vi "RIS.vi"(2 "Run uninterrupted?":bool, 3 "Device Category IN:":string(combo)="Short Strip" caption="Device Category:", 4 "Batch No.:":string, 5 "Wafer Serial No.:":string, 6 "Sensor Serial No.:":string) -> (0 "Done!":bool)   [LabVIEW 2018]
doc: "Performs Ris measurements according to ATLAS ITk Quality Control Specifications."
uses:
  <vilib>/Analysis/6fits.llb/Curve Fitting Criteria.ctl
  general_VIs/globals/QC_MeasurementSetup.vi
  general_VIs/globals/QC_RunInformation.vi
  InstrControl/InstrumentSetup.vi
  InstrControl/Switching/Switching.lvclass
  InstrControl/SupplyControl/SupplyControl.lvclass
  InstrControl/MultimeterControl/MultimeterControl.lvclass
  InstrControl/ArduinoControl/ArduinoControl.lvclass
  <vilib>/Analysis/NI_AALBase.lvlib
  InstrControl/InstrControl.lvclass
  <vilib>/Analysis/NI_AALPro.lvlib
panel:
  out "Ris":dbl[](array[numeric]) caption="Ris [MOhm]"
  out "Volts":dbl[](array[numeric]) caption="Volts [V]"
  out "Current":dbl[](array[numeric]) caption="Current [nA]"
  in  "No. of readouts":i32=5
  out "Risgraph":cluster{dbl[], dbl[]}(graph)
  out "Vigraph":cluster{i32[], dbl[]}[](graph)
  out "Imgraph":cluster{i32[], dbl[]}[](graph)
  out "Initial volts [V]":dbl format="%.1f"
  out "Final volts [V]":dbl=-700.0 format="%.1f"
  out "step [V]":dbl=10.0 format="%.1f"
  out "step interval [s]":u32=10
  out "Temp.":dbl[](array[numeric]) caption="Temp. [°C]" format="%#.2f"
  out "RH":dbl[](array[numeric]) caption="RH [%]" format="%#.2f"
  out "positive ramp?":bool
  out "Tab Control":enum32{"Ris Setup", "Ris Scan"}(tab)
  in  "Voltmeter":string(combo)="Keithley 2410"
  in  "Ris SMU":string(combo)="Keithley 2410"
  in  "Current \nLimit \n[µA]":dbl=1000.0 min=0.0001 format="%.3f"
  in  "Set\ncurrent\nlimit?":bool
  in  "Temperature":enum16{"Read Arduino", "Enter manually"}(ring)
  in  "Ris Supply":string(combo)="Keithley 2410"
  in  "User:":string(combo)="Christoph"
  in  "Configurations":bool
  in  "Manufacturer:":string(combo)="Hamamatsu"
  in  "Quit":bool
  in  "Continue":bool
  in  "abort":bool
  out "Device Category:":string
  out "Batch:":string
  out "Current Volts:":dbl format="%.2f"
  in  "quit (no save)":bool
  in  "Quit & Save":bool
  out "Bias On/Off:":bool
  out "STATUS 1":string
  out "Initiated:":string
  out "Sensor No.:":string
  out "No of steps":u32
  out "Current reading No.":u32
  out "Last reading at:":string
  out "Ris SMU Current [nA]":dbl[][][](array[numeric])
  out "Ris induced Voltage [V]":dbl[][][](array[numeric])
  # "University of\nCambridge"
  # "Strip Sensor QC: inter-strip Resistance"
  # "Ris Scan parameters:"
  # "Last 5 readings:"
  # "n-4"
  # "n-3"
  # "n-2"
  # "n-1"
  # "n"
  # "DUT & Test Description"
  # "Hardware"
  # "DUT & Test Description:"
  # "Current status:"
  # "Rdg No:"
  # "out of"
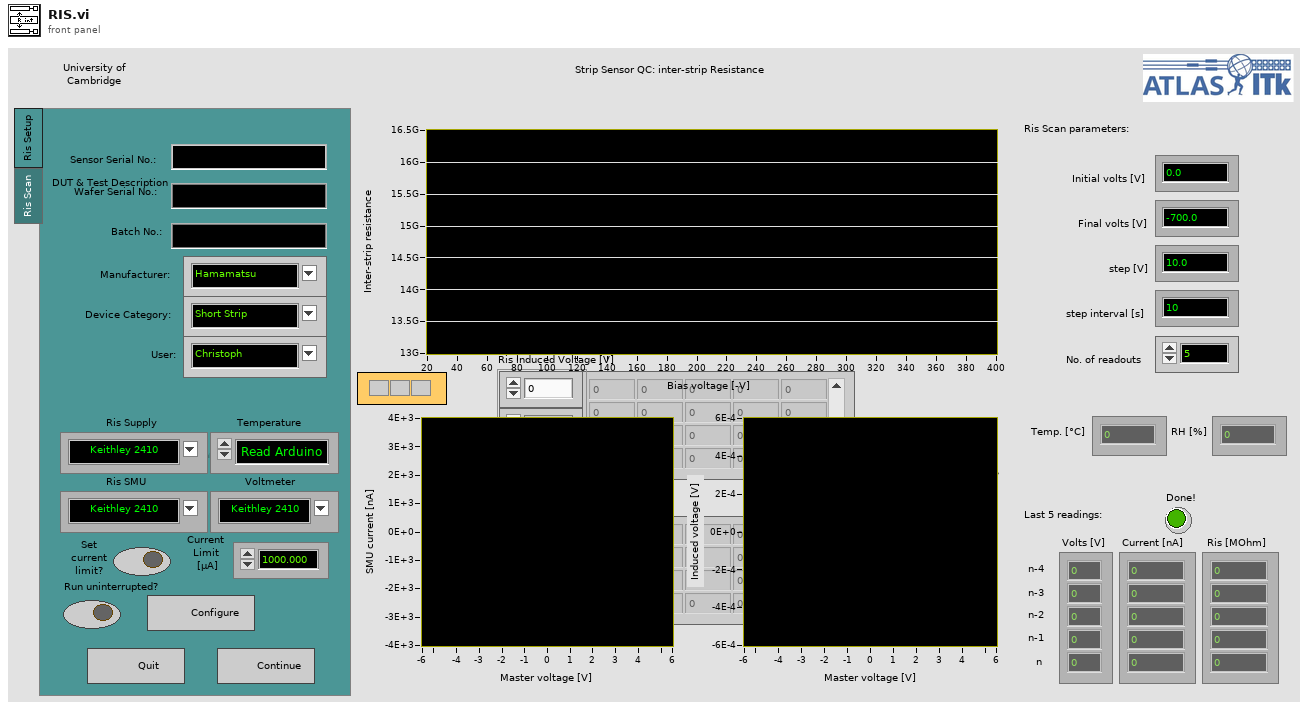
[diagram p1: front panel]
types:
  T1 = enum16{"Supply", "LCR", "Multimeter", "Switching"}
  T2 = enum16{"Reset", "Read Array", "Read Element", "Write Element", "Write Array", "Add Element", "Add Array"}
  T3 = enum16{"Reset", "Ground", "Striptest SMU", "Striptest LCR", "IV", "CV", "Interstrip Cap", "Interstrip Res"}
  T4 = enum32{"IV", "CV", "Stability", "Striptest", "Cis", "Ris", "PTP"}
  T5 = cluster{"Sensor Serial No.:":string, "Wafer Serial No.:":string, "Batch:":string, "Manufacturer:":string, "Device Category:":string, "Database Serial No.:":string, "Date Initiated:":string, "Time Initiated:":string, "Test":string, "Instruments used:":string, "Probeplan used:":string, "End of Run comment:":string, "User:":string}
  T6 = cluster{"Institute":string, "Manufacturers":string[], "Devices":string[], "Serialnumbers Lookup DB":string, "Data directory":string, "Backup & screenshot directory":string, "List of known users":string[], "Measurement switch not used":bool, "Measurement Switch":string, "DUT Switch":string}
  T7 = cluster{"Bias Supply":refnum<class "SupplyControl.lvclass">, "SMU":refnum<class "SupplyControl.lvclass">, "Multimeter":refnum<class "MultimeterControl.lvclass">, "Initial Voltage [V]":dbl, "Final Voltage [V]":dbl, "Step Size [V]":dbl, "Step Interval [s]":i32, "Number Of Steps":u32, "Ramp down steps [V]":dbl, "Ramp down Interval [s]":i32, "Set Current Limit?":bool, "Current Limit [µA]":dbl, "Temperature Readout":enum16{"Read Arduino", "Enter manually"}, "Arduino":refnum<class "ArduinoControl.lvclass">, "Supply Name":string, "SMU Name":string, "Voltmeter Name":string, "R_is Limit [MOhm]":dbl, "Switching":refnum<class "Switching.lvclass">, "Matrix used?":bool, "Matrix X Channels":cluster{"Bias Supply / SMU LO":i32, "Bias Supply / SMU HI":i32, "CV Box LO":i32, "CV Box HI":i32, "CV Box LO IN":i32, "CV Box HI IN":i32, "Volt meter LO":i32, "Volt meter HI":i32, "Mux1 C1":i32, "Mux1 C2":i32, "Mux2 C1":i32, "Mux2 C2":i32}}
  T8 = cluster{"VISA address":refnum<visa-resource-name>, "T sensor":enum16{"SHT", "DS"}, "Arduino":refnum<class "ArduinoControl.lvclass">}
  T9 = typedef "NI_AALPro.lvlib/Curve Fitting Criteria.ctl" = u16
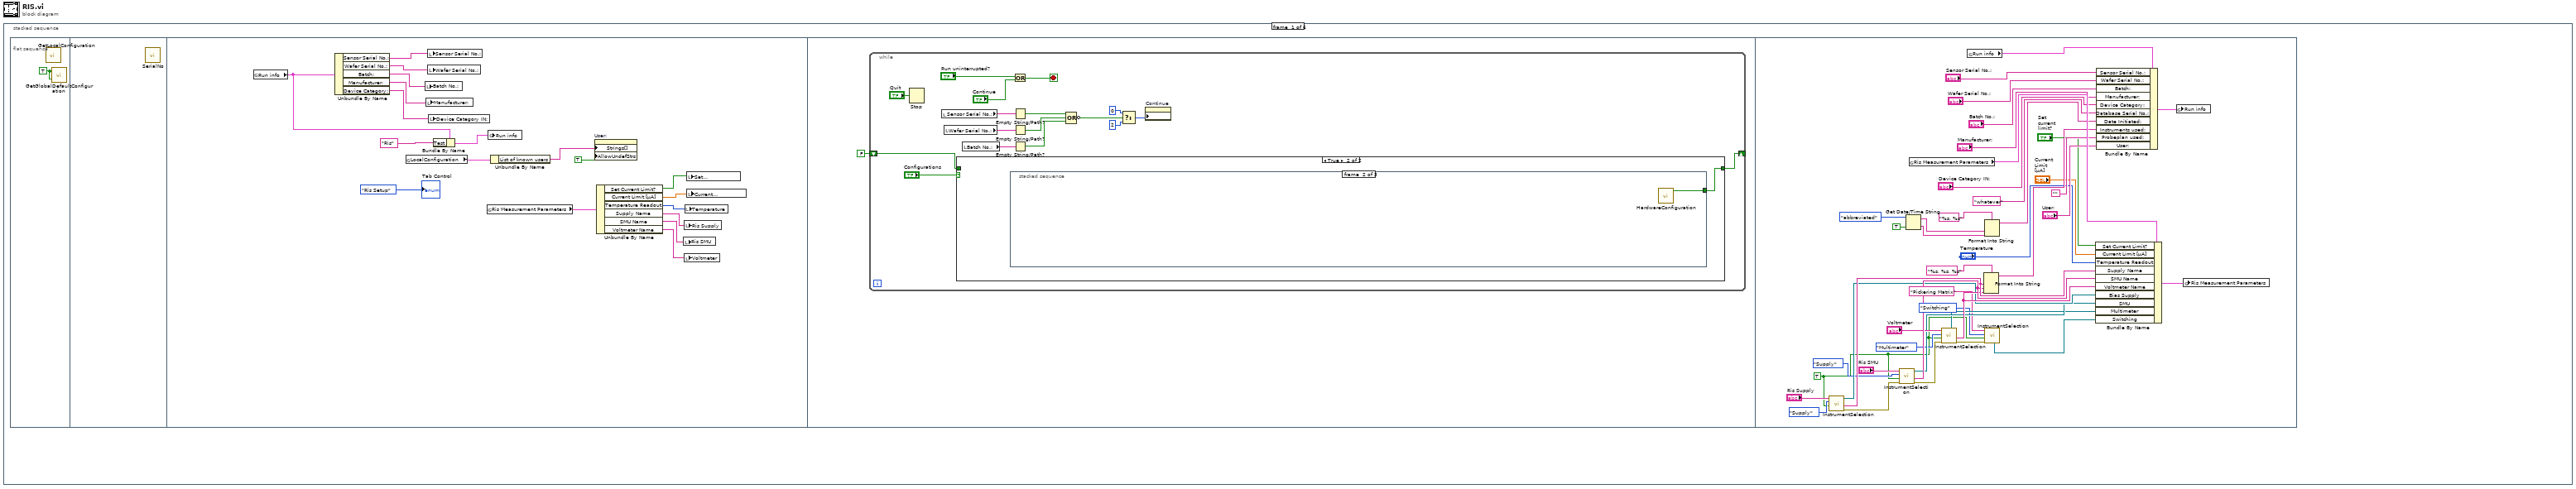
[diagram p0: block diagram]
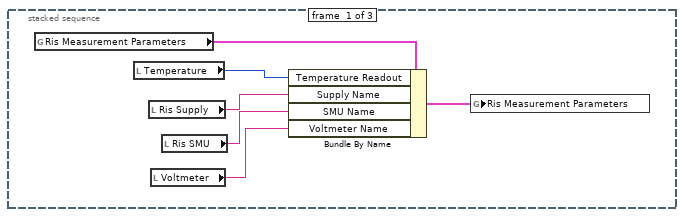
[diagram p3: hidden frame]
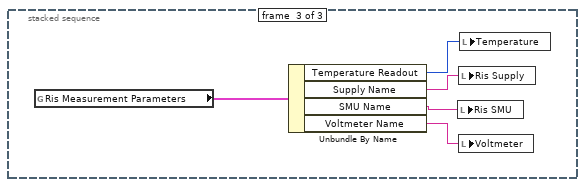
[diagram p4: hidden frame]
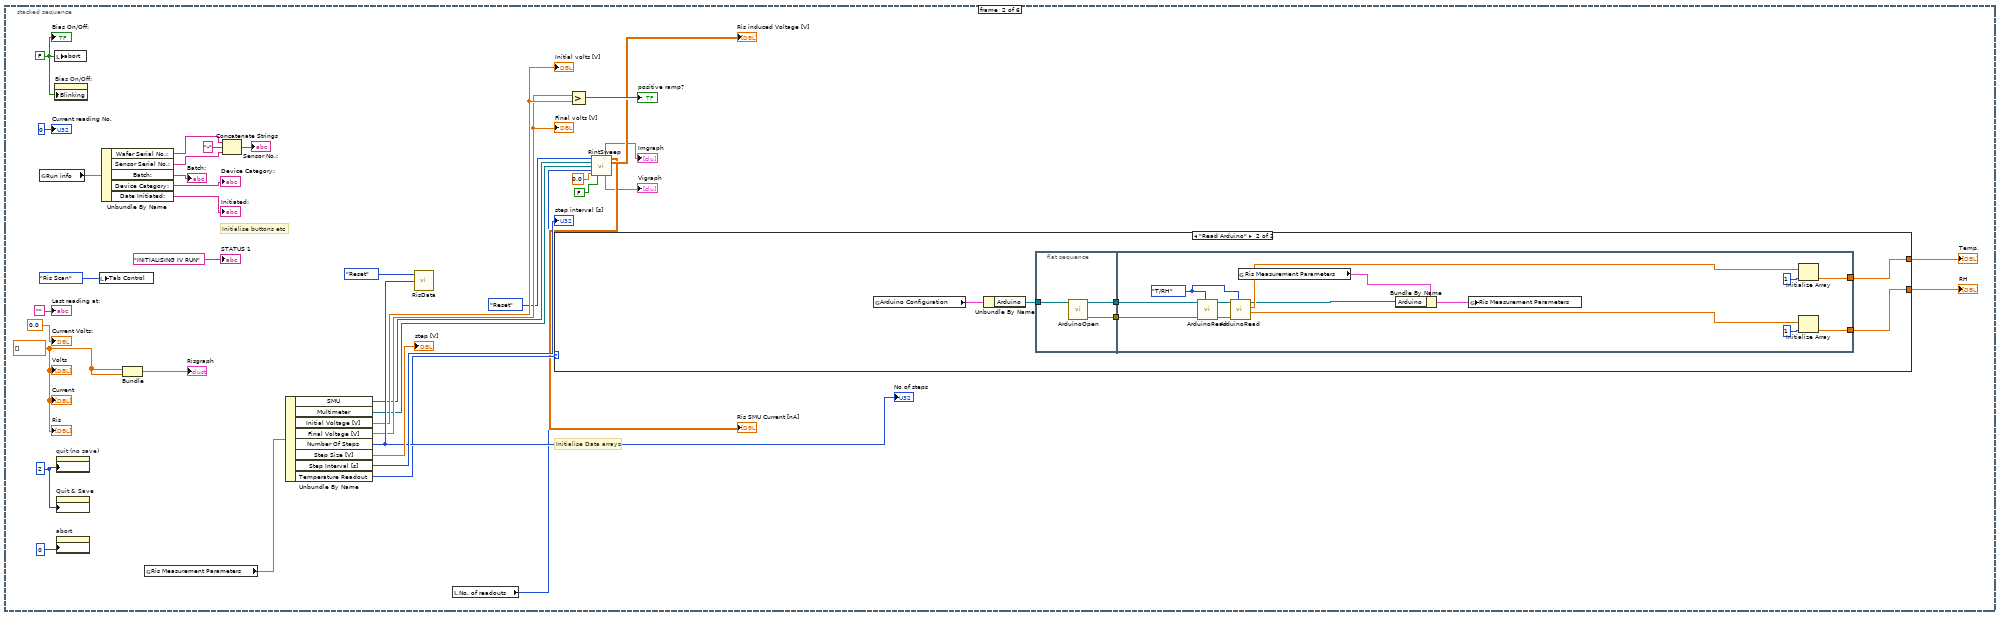
[diagram p5: hidden frame]
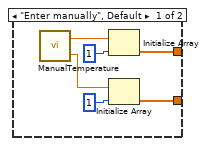
[diagram p6: hidden frame]
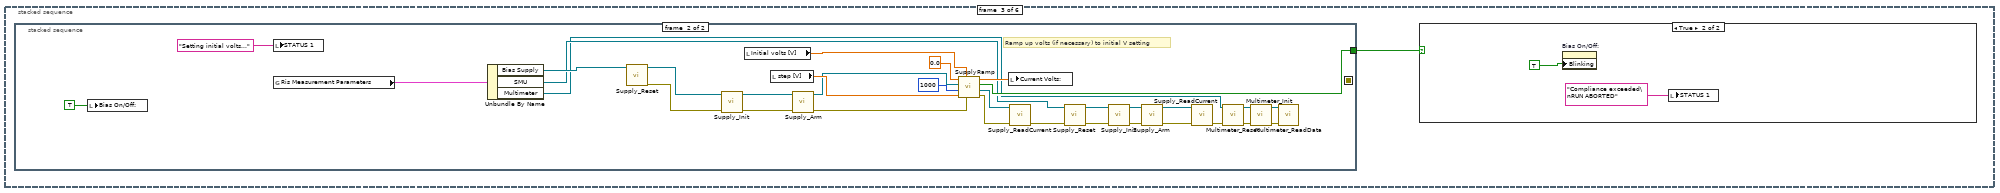
[diagram p7: hidden frame]
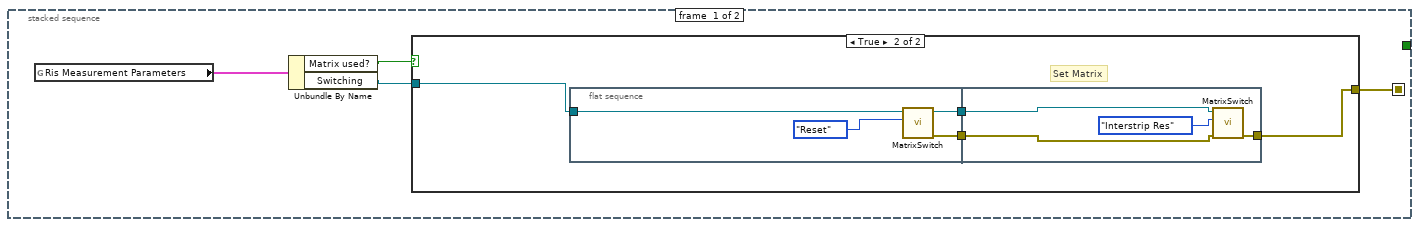
[diagram p8: hidden frame]
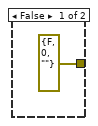
[diagram p9: hidden frame]
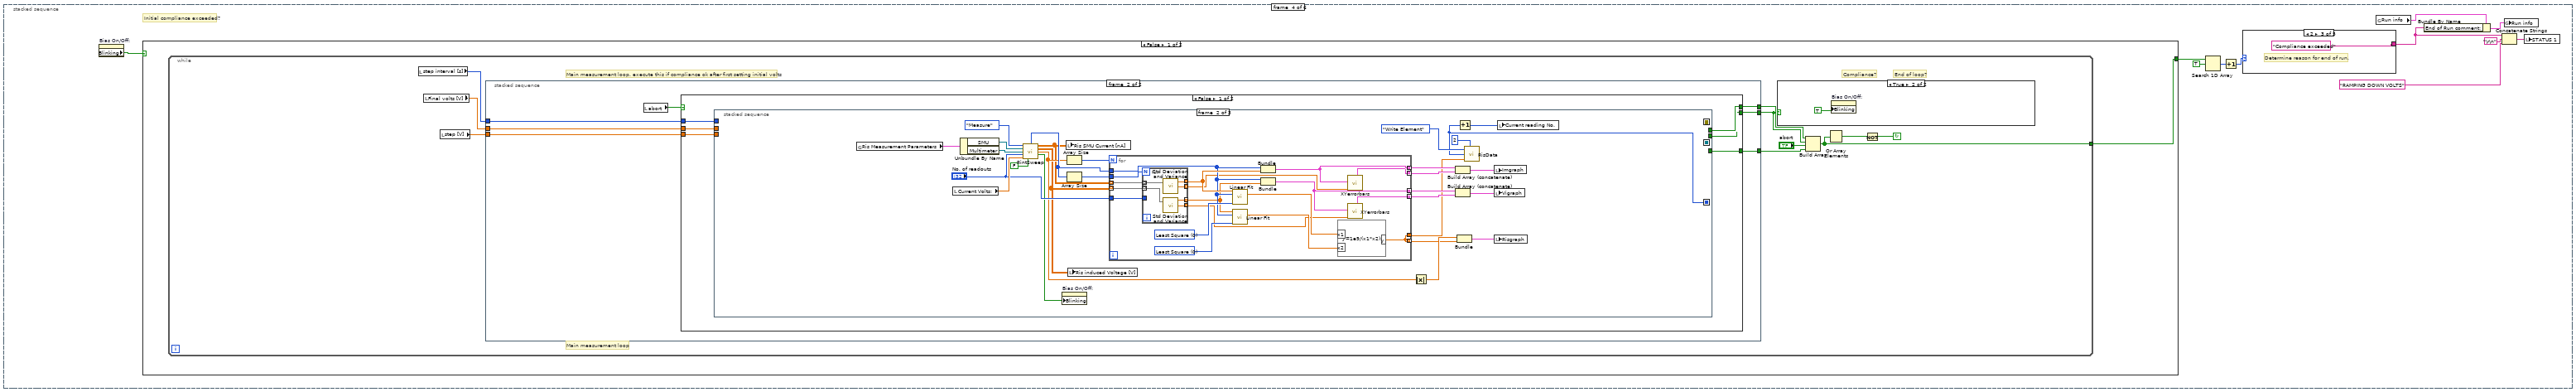
[diagram p11: hidden frame]
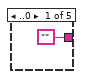
[diagram p12: hidden frame]
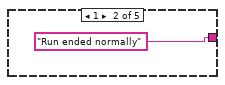
[diagram p13: hidden frame]
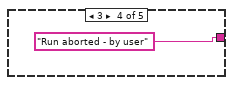
[diagram p14: hidden frame]
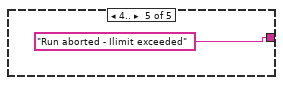
[diagram p15: hidden frame]
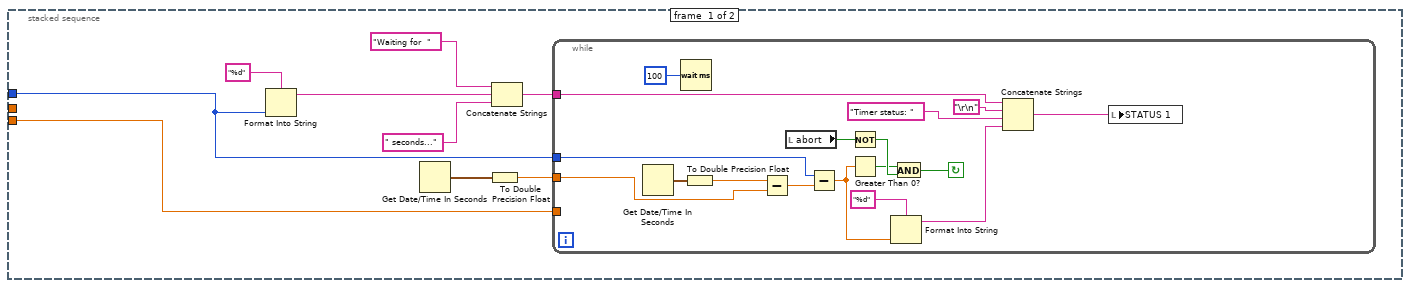
[diagram p16: hidden frame]
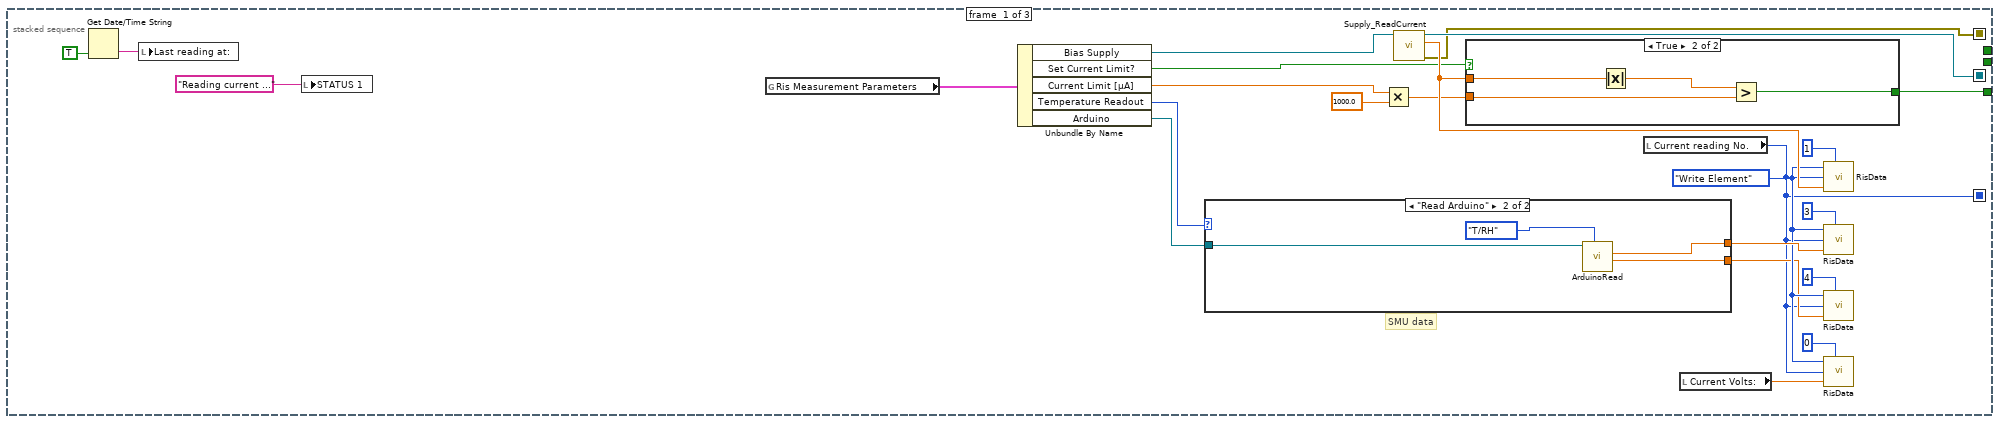
[diagram p17: hidden frame]
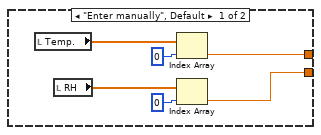
[diagram p18: hidden frame]
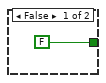
[diagram p19: hidden frame]
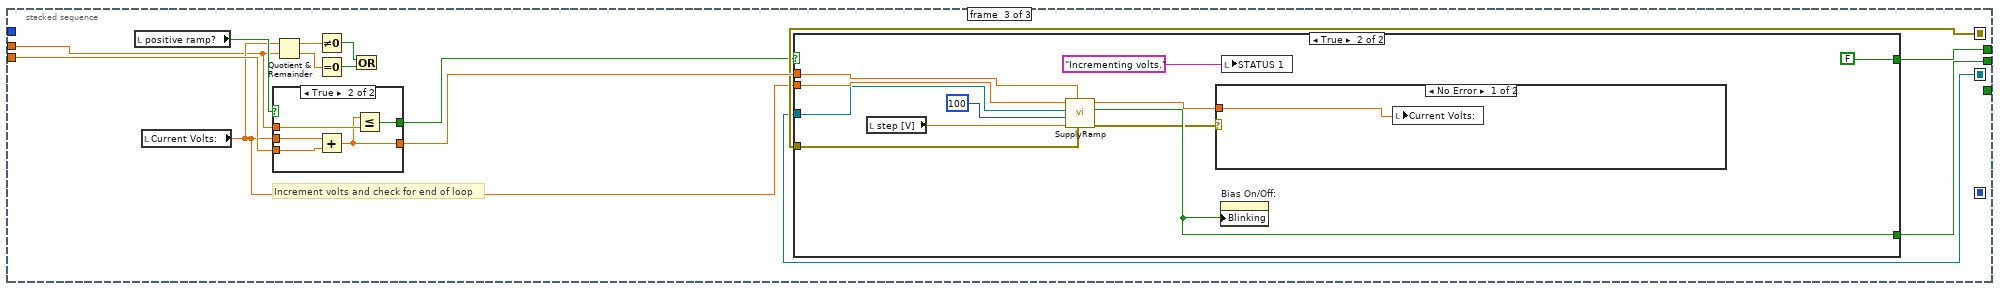
[diagram p20: hidden frame]
diagram:
  n1 = stacked-sequence {
    frame #0 {
      n2 = flat-sequence {
        frame #0 {
          w1 = TRUE
          n3 = call "GetLocalConfiguration.vi"() -> ()  [unwired: 3 in, 1 out]
          n4 = call "GetGlobalDefaultConfiguration.vi"("Run uninterrupted"=w1, "Read defaults?"=w1) -> ()  [unwired: 1 in, 1 out]
        }
        frame #1 {
          n5 = call "SerialNo.vi"() -> ()  [unwired: 5 in, 1 out]
        }
        frame #2 {
          n6 = global read "QC_RunInformation.vi" "Run info"() -> (w7:T5)
          n7 = Unbundle By Name(w7) -> ("Sensor Serial No.:"=w3:string, "Wafer Serial No.:"=w4:string, "Batch:"=w5:string, "Manufacturer:"=w2:string, "Device Category:"=w6:string)
          n8 = global read "QC_RunInformation.vi" "LocalConfiguration"() -> (w15:T6)
          n9 = local write "Batch No.:"(w5) -> ()
          n10 = local write "Manufacturer:"(w2) -> ()
          n11 = local write "Sensor Serial No.:"(w3) -> ()
          n12 = local write "Wafer Serial No.:"(w4) -> ()
          n13 = local write "Device Category IN:"(w6) -> ()
          n14 = Bundle By Name(cluster=w7, "Test"="Ris") -> (w12:T5)
          n15 = global read "QC_MeasurementSetup.vi" "Ris Measurement Parameters"() -> (w18:T7)
          n16 = global write "QC_RunInformation.vi" "Run info"(w12) -> ()
          n17 = Unbundle By Name(w15) -> ("List of known users"=w14:string[])
          n18 = property on="User:" class="CmbBox"("Strings[]"=w14, "AllowUndefStrs"=TRUE) -> ()  [unwired: 2 in, 2 out]
          n19 = Unbundle By Name(w18) -> ("Set Current Limit?"=w17:bool, "Current Limit [µA]"=w16:dbl, "Temperature Readout"=w20:enum16{"Read Arduino", "Enter manually"}, "Supply Name"=w19:string, "SMU Name"=w9:string, "Voltmeter Name"=w8:string)
          n20 = local write "Ris SMU"(w9) -> ()
          n21 = local write "Ris Supply"(w19) -> ()
          n22 = local write "Voltmeter"(w8) -> ()
          n23 = local write "Temperature"(w20) -> ()
          n24 = local write "Set\ncurrent\nlimit?"(w17) -> ()
          n25 = local write "Current \nLimit \n[µA]"(w16) -> ()
          "Tab Control" <- enum32{"Ris Setup", "Ris Scan"}."Ris Setup" ("Tab Control")
        }
        frame #3 {
          n26 = while {
            shift-right: [w26] -> _
            shift-left: FALSE -> [w25]
            stop <- w22 stop-if-true
            n27 = Stop(stop? (T)="Quit") -> ()
            n28 = local read "Sensor Serial No.:"() -> (w37:string)
            n29 = local read "Wafer Serial No.:"() -> (w36:string)
            n30 = case shown="True" "Configurations" {
              tunnel: [w39 w40] -> w26
              tunnel: w25 -> [w39 _]
              frame False {
              }
              frame True {
                n31 = stacked-sequence {
                  tunnel: [_ w47 _] -> w40
                  frame #0 {
                    n32 = global read "QC_MeasurementSetup.vi" "Ris Measurement Parameters"() -> (w46:T7)
                    n33 = local read "Temperature"() -> (w45:enum16{"Read Arduino", "Enter manually"})
                    n34 = local read "Ris Supply"() -> (w44:string)
                    n35 = local read "Voltmeter"() -> (w42:string)
                    n36 = local read "Ris SMU"() -> (w43:string)
                    n37 = Bundle By Name(cluster=w46, "Temperature Readout"=w45, "Supply Name"=w44, "SMU Name"=w43, "Voltmeter Name"=w42) -> (w41:T7)
                    n38 = global write "QC_MeasurementSetup.vi" "Ris Measurement Parameters"(w41) -> ()
                  }
                  frame #1 {
                    n39 = call "HardwareConfiguration.vi"() -> ("configured?"=w47:bool)  [unwired: 11 in]
                  }
                  frame #2 {
                    n40 = global read "QC_MeasurementSetup.vi" "Ris Measurement Parameters"() -> (w52:T7)
                    n41 = Unbundle By Name(w52) -> ("Temperature Readout"=w48:enum16{"Read Arduino", "Enter manually"}, "Supply Name"=w49:string, "SMU Name"=w50:string, "Voltmeter Name"=w51:string)
                    n42 = local write "Ris SMU"(w50) -> ()
                    n43 = local write "Ris Supply"(w49) -> ()
                    n44 = local write "Voltmeter"(w51) -> ()
                    n45 = local write "Temperature"(w48) -> ()
                  }
                }
              }
            }
            n46 = local read "Batch No.:"() -> (w28:string)
            n47 = Or(x="Run uninterrupted?", y="Continue") -> (x .or. y?=w22:bool)
            n48 = Empty String/Path?(string/path=w37) -> (empty?=w34:bool)
            n49 = Empty String/Path?(string/path=w36) -> (empty?=w35:bool)
            n50 = Empty String/Path?(string/path=w28) -> (empty?=w27:bool)
            n51 = Compound Arithmetic op=OR(w34, w35, w27) -> (invert w33:bool)
            n52 = Select(t=0, s=w33, f=2) -> (s? t:f=w30:i32)
            n53 = property on="Continue" class="Bool"("DisabledEnum"=w30) -> ()  [unwired: 2 in, 2 out]
          }
        }
        frame #4 {
          w55 = TRUE
          n54 = call "InstrumentSelection.vi"("Verify GPIB address"=w55, "Instrument type"=T1."Supply", "Instrument name IN"="Ris Supply") -> ("error out"=w62:errorcluster, "Instrument name OUT"=w70:string, "Supply"=w65:refnum<class "SupplyControl.lvclass">)  [unwired: 3 in, 3 out]
          n55 = call "InstrumentSelection.vi"("error in (no error)"=w62, "Verify GPIB address"=w55, "Instrument type"=T1."Supply", "Instrument name IN"="Ris SMU") -> ("error out"=w61:errorcluster, "Instrument name OUT"=w68:string, "Supply"=w64:refnum<class "SupplyControl.lvclass">)  [unwired: 2 in, 3 out]
          n56 = Get Date/Time String(date format (0)=enum16{"short", "long", "abbreviated"}."abbreviated", want seconds? (F)=TRUE) -> (date string=w90:string, time string=w89:string)  [unwired: 1 in]
          n57 = global read "QC_MeasurementSetup.vi" "Ris Measurement Parameters"() -> (w93:T7)
          n58 = call "InstrumentSelection.vi"("error in (no error)"=w61, "Verify GPIB address"=w55, "Instrument type"=T1."Multimeter", "Instrument name IN"="Voltmeter") -> ("error out"=w60:errorcluster, "Instrument name OUT"=w66:string, "Multimeter"=w63:refnum<class "MultimeterControl.lvclass">)  [unwired: 2 in, 3 out]
          n59 = global read "QC_RunInformation.vi" "Run info"() -> (w87:T5)
          n60 = Format Into String(format string="%s, %s, %s", w70, w68, w66) -> (resulting string=w75:string)  [unwired: 2 in, 1 out]
          n61 = Format Into String(format string="%s, %s", w90, w89) -> (resulting string=w85:string)  [unwired: 2 in, 1 out]
          n62 = call "InstrumentSelection.vi"("error in (no error)"=w60, "Verify GPIB address"=w55, "Instrument type"=T1."Switching", "Instrument name IN"="Pickering Matrix") -> ("Switching"=w54:refnum<class "Switching.lvclass">)  [unwired: 2 in, 5 out]
          n63 = Bundle By Name(cluster=w93, "Set Current Limit?"="Set\ncurrent\nlimit?", "Current Limit [µA]"="Current \nLimit \n[µA]", "Temperature Readout"="Temperature", "Supply Name"=w70, "SMU Name"=w68, "Voltmeter Name"=w66, "Bias Supply"=w65, "SMU"=w64, "Multimeter"=w63, "Switching"=w54) -> (w94:T7)
          n64 = Bundle By Name(cluster=w87, "Sensor Serial No.:"="Sensor Serial No.:", "Wafer Serial No.:"="Wafer Serial No.:", "Batch:"="Batch No.:", "Manufacturer:"="Manufacturer:", "Device Category:"="Device Category IN:", "Database Serial No.:"="whatever", "Date Initiated:"=w85, "Instruments used:"=w75, "Probeplan used:"="", "User:"="User:") -> (w86:T5)
          n65 = global write "QC_RunInformation.vi" "Run info"(w86) -> ()
          n66 = global write "QC_MeasurementSetup.vi" "Ris Measurement Parameters"(w94) -> ()
        }
      }
    }
    frame #1 {
      w100 = dbl[] []
      w122 = 2
      w121 = FALSE ("Visible")
      # "Initialise buttons etc"
      # "Initialise Data arrays"
      n67 = global read "QC_RunInformation.vi" "Run info"() -> (w132:T5)
      n68 = local write "abort"(w121) -> ()
      n69 = property on="Bias On/Off:" class="Bool (strict)"("Blinking"=w121) -> ()  [unwired: 2 in, 2 out]
      n70 = property on="quit (no save)" class="Bool"("DisabledEnum"=w122) -> ()  [unwired: 2 in, 2 out]
      n71 = property on="Quit & Save" class="Bool"("DisabledEnum"=w122) -> ()  [unwired: 2 in, 2 out]
      n72 = property on="abort" class="Bool (strict)"("DisabledEnum"=0) -> ()  [unwired: 2 in, 2 out]
      n73 = local write "Tab Control"(enum32{"Ris Setup", "Ris Scan"}."Ris Scan" ("Tab Control")) -> ()
      n74 = Unbundle By Name(w132) -> ("Wafer Serial No.:"=w113:string, "Sensor Serial No.:"=w112:string, "Batch:"=→"Batch:":string, "Device Category:"=→"Device Category:":string, "Date Initiated:"=→"Initiated:":string)
      n75 = Bundle(w100, w100) -> (→"Risgraph":cluster{dbl[], dbl[]})  [unwired: 1 in]
      n76 = global read "QC_MeasurementSetup.vi" "Ris Measurement Parameters"() -> (w115:T7)
      n77 = Concatenate Strings(w113, "-", w112) -> (→"Sensor No.:":string)
      n78 = Unbundle By Name(w115) -> ("SMU"=w96:refnum<class "SupplyControl.lvclass">, "Multimeter"=w95:refnum<class "MultimeterControl.lvclass">, "Initial Voltage [V]"=w120:dbl, "Final Voltage [V]"=w119:dbl, "Number Of Steps"=w128:u32, "Step Size [V]"=→"step [V]":dbl, "Step Interval [s]"=→"step interval [s]":i32, "Temperature Readout"=w123:enum16{"Read Arduino", "Enter manually"})
      "No of steps" <- w128
      "Initial volts [V]" <- w120
      "Final volts [V]" <- w119
      n79 = call "RisData.vi"("Action"=T2."Reset", "Array Size / Index"=w128) -> ()  [unwired: 3 in, 2 out]
      n80 = local read "No. of readouts"() -> (w98:i32)
      n81 = case shown="\"Read Arduino\"" w123 {
        tunnel: [w138 w145] -> w125
        tunnel: [w135 w144] -> w116
        frame "Enter manually", Default {
          n82 = call "ManualTemperature.vi"() -> ("Humidity [%] out"=w134:dbl, "Temperature [°C] out"=w139:dbl)
          n83 = Initialize Array(w139, 1) -> (w138:dbl[])
          n84 = Initialize Array(w134, 1) -> (w135:dbl[])
        }
        frame "Read Arduino" {
          n85 = global read "InstrumentSetup.vi" "Arduino Configuration"() -> (w141:T8)
          n86 = Unbundle By Name(w141) -> ("Arduino"=w140:refnum<class "ArduinoControl.lvclass">)
          n87 = flat-sequence {
            tunnel: [w146] -> w143
            tunnel: [w148] -> w142
            tunnel: w140 -> [w147]
            tunnel: [w162] -> w145
            tunnel: [w159] -> w144
            tunnel: w143 -> [w153]
            tunnel: w142 -> [w152]
            frame #0 {
              n88 = call "ArduinoOpen.vi"("ArduinoControl in"=w147) -> ("error out"=w148:errorcluster, "ArduinoControl out"=w146:refnum<class "ArduinoControl.lvclass">)  [unwired: 9 in]
            }
            frame #1 {
              w149 = enum16{"T/RH", "Interlock", "Edgesense"}."T/RH" ("Arduino function")
              n89 = call "ArduinoRead.vi"("Arduino function"=w149, "error in (no error)"=w152, "ArduinoControl in"=w153) -> ("error out"=w151:errorcluster, "ArduinoControl out"=w150:refnum<class "ArduinoControl.lvclass">)  [unwired: 3 in, 4 out]
              n90 = call "ArduinoRead.vi"("Arduino function"=w149, "error in (no error)"=w151, "ArduinoControl in"=w150) -> ("rel. Humidity [%]"=w157:dbl, "Temperature [°C]"=w158:dbl, "ArduinoControl out"=w156:refnum<class "ArduinoControl.lvclass">)  [unwired: 3 in, 3 out]
              n91 = global read "QC_MeasurementSetup.vi" "Ris Measurement Parameters"() -> (w155:T7)
              n92 = Bundle By Name(cluster=w155, "Arduino"=w156) -> (w154:T7)
              n93 = global write "QC_MeasurementSetup.vi" "Ris Measurement Parameters"(w154) -> ()
              n94 = Initialize Array(w158, 1) -> (w162:dbl[])
              n95 = Initialize Array(w157, 1) -> (w159:dbl[])
            }
          }
        }
      }
      "Temp." <- w125
      "RH" <- w116
      n96 = Greater?(x=w119, y=w120) -> (0:→"positive ramp?":bool)
      n97 = call "RintSweep.vi"("Action"=enum16{"Reset", "Measure"}."Reset", "MasterVoltage Supply in"=w96, "VoltmeterControl in"=w95, "No. of readouts"=w98, "Bias [V]"=0.0, "Simulated data?"=FALSE) -> ("Igraph"=→"Imgraph":cluster{i32[], dbl[]}[], "Applied Current [nA]"=→"Ris SMU Current [nA]":dbl[][][], "Induced Voltage [V]"=→"Ris induced Voltage [V]":dbl[][][], "ViGraph"=→"Vigraph":cluster{i32[], dbl[]}[])  [unwired: 2 in, 4 out]
      "STATUS 1" <- "INITIALISING IV RUN"
      "Bias On/Off:" <- w121
      "Last reading at:" <- ""
      "Current reading No." <- u32 0 ("Current reading No.")
      "Current Volts:" <- 0.0 ("Current Volts:")
      "Current" <- w100
      "Volts" <- w100
      "Ris" <- w100
    }
    frame #2 {
      n98 = stacked-sequence {
        seq-local: [w165 _] -> [_ _]
        tunnel: [_ w195] -> w163
        frame #0 {
          n99 = global read "QC_MeasurementSetup.vi" "Ris Measurement Parameters"() -> (w164:T7)
          n100 = Unbundle By Name(w164) -> ("Matrix used?"=w167:bool, "Switching"=w166:refnum<class "Switching.lvclass">)
          n101 = case shown="True" w167 {
            tunnel: w166 -> [_ w169]
            tunnel: [errorcluster {"status"=FALSE, "code"=0, "source"=""} ("error constant") w170] -> w165
            frame False {
            }
            frame True {
              # "Set Matrix"
              n102 = flat-sequence {
                tunnel: [w176] -> w172
                tunnel: [w175] -> w171
                tunnel: w169 -> [w173]
                tunnel: w172 -> [w180]
                tunnel: w171 -> [w179]
                tunnel: [w178] -> w170
                frame #0 {
                  n103 = call-dynamic "MatrixSwitch.vi"("Action"=T3."Reset", "Switching in"=w173) -> ("error out"=w176:errorcluster, "Switching out"=w175:refnum<class "Switching.lvclass">)  [unwired: 7 in, 1 out]
                }
                frame #1 {
                  n104 = call-dynamic "MatrixSwitch.vi"("error in (no error)"=w180, "Action"=T3."Interstrip Res", "Switching in"=w179) -> ("error out"=w178:errorcluster)  [unwired: 6 in, 2 out]
                }
              }
            }
          }
        }
        frame #1 {
          # "Ramp up volts (if necessary) to initial V setting"
          n105 = local write "Bias On/Off:"(TRUE ("Compliance?")) -> ()
          n106 = local write "STATUS 1"("Setting initial volts..." ("STATUS 1")) -> ()
          n107 = global read "QC_MeasurementSetup.vi" "Ris Measurement Parameters"() -> (w208:T7)
          n108 = Unbundle By Name(w208) -> ("Bias Supply"=w205:refnum<class "SupplyControl.lvclass">, "SMU"=w187:refnum<class "SupplyControl.lvclass">, "Multimeter"=w182:refnum<class "MultimeterControl.lvclass">)
          n109 = call-dynamic "Supply_Reset.vi"("SupplyControl in"=w205) -> ("error out"=w210:errorcluster, "SupplyControl out"=w212:refnum<class "SupplyControl.lvclass">)  [unwired: 9 in]
          n110 = call-dynamic "Supply_Init.vi"("error in (no error)"=w210, "SupplyControl in"=w212) -> ("error out"=w209:errorcluster, "SupplyControl out"=w211:refnum<class "SupplyControl.lvclass">)  [unwired: 8 in]
          n111 = local read "Initial volts [V]"() -> (w198:dbl)
          n112 = local read "step [V]"() -> (w199:dbl)
          n113 = call-dynamic "Supply_Arm.vi"("error in (no error)"=w209, "SupplyControl in"=w211) -> ("error out"=w197:errorcluster, "SupplyControl out"=w196:refnum<class "SupplyControl.lvclass">)  [unwired: 8 in]
          n114 = call "SupplyRamp.vi"("error in"=w197, "Requested Voltage"=w198, "Step Size"=w199, "Step Delay"=1000, "Supply IN"=w196, "Starting Voltage"=0.0) -> ("error out"=w203:errorcluster, "Supply OUT"=w204:refnum<class "SupplyControl.lvclass">, "Compliance exceeded"=w195:bool, "Current Voltage"=w202:dbl)  [unwired: 2 in]
          n115 = local write "Current Volts:"(w202) -> ()
          n116 = call-dynamic "Supply_ReadCurrent.vi"("error in (no error)"=w203, "SupplyControl in"=w204) -> ("error out"=w188:errorcluster)  [unwired: 7 in, 2 out]
          n117 = call-dynamic "Supply_Reset.vi"("error in (no error)"=w188, "SupplyControl in"=w187) -> ("error out"=w192:errorcluster, "SupplyControl out"=w194:refnum<class "SupplyControl.lvclass">)  [unwired: 8 in]
          n118 = call-dynamic "Supply_Init.vi"("error in (no error)"=w192, "SupplyControl in"=w194) -> ("error out"=w191:errorcluster, "SupplyControl out"=w193:refnum<class "SupplyControl.lvclass">)  [unwired: 8 in]
          n119 = call-dynamic "Supply_Arm.vi"("error in (no error)"=w191, "SupplyControl in"=w193) -> ("error out"=w190:errorcluster, "SupplyControl out"=w189:refnum<class "SupplyControl.lvclass">)  [unwired: 8 in]
          n120 = call-dynamic "Supply_ReadCurrent.vi"("error in (no error)"=w190, "SupplyControl in"=w189) -> ("error out"=w181:errorcluster)  [unwired: 7 in, 2 out]
          n121 = call-dynamic "Multimeter_Reset.vi"("error in (no error)"=w181, "MultimeterControl in"=w182) -> ("error out"=w183:errorcluster, "MultimeterControl out"=w184:refnum<class "MultimeterControl.lvclass">)  [unwired: 8 in]
          n122 = call-dynamic "Multimeter_Init.vi"("error in (no error)"=w183, "MultimeterControl in"=w184) -> ("error out"=w186:errorcluster, "MultimeterControl out"=w185:refnum<class "MultimeterControl.lvclass">)  [unwired: 8 in]
          n123 = call-dynamic "Multimeter_ReadData.vi"("error in (no error)"=w186, "MultimeterControl in"=w185) -> ()  [unwired: 7 in, 3 out]
        }
      }
      n124 = case shown="True" w163 {
        frame False {
        }
        frame True {
          n125 = property on="Bias On/Off:" class="Bool (strict)"("Blinking"=TRUE) -> ()  [unwired: 2 in, 2 out]
          n126 = local write "STATUS 1"("Compliance exceeded\nRUN ABORTED") -> ()
        }
      }
    }
    frame #3 {
      # "Initial compliance exceeded?"
      n127 = property on="Bias On/Off:" class="Bool (strict)"() -> ("Blinking"=w225:bool)  [unwired: 2 in, 2 out]
      n128 = case shown="False" w225 {
        tunnel: [w231 w413] -> w224
        frame False {
          n129 = while {
            tunnel: [w239] -> w231
            stop <- w240 continue-if-true
            # "Main measurement loop"
            # "End of loop?"
            # "Compliance?"
            # "Main measurement loop. execute this if compliance ok after first setting initial volts"
            n130 = local read "step interval [s]"() -> (w236:u32)
            n131 = local read "Final volts [V]"() -> (w237:dbl)
            n132 = local read "step [V]"() -> (w238:dbl)
            n133 = stacked-sequence {
              tunnel: w238 -> [w250 w274]
              tunnel: [_ w273] -> w233
              tunnel: w237 -> [_ w272]
              tunnel: w236 -> [w242 w271]
              tunnel: [_ w270] -> w235
              tunnel: [_ w268] -> w234
              frame #0 {
                n134 = Format Into String(format string="%d", w242) -> (resulting string=w247:string)  [unwired: 2 in, 1 out]
                n135 = Get Date/Time In Seconds() -> (seconds since 1Jan1904=w244:timestamp)
                n136 = To Double Precision Float(number=w244) -> (double precision float=w245:dbl)
                n137 = Concatenate Strings("Waiting for  ", w247, " seconds...") -> (w243:string)
                n138 = while {
                  tunnel: w250 -> [_]
                  tunnel: w243 -> [w255]
                  tunnel: w242 -> [w261]
                  tunnel: w245 -> [w262]
                  stop <- w263 continue-if-true
                  n139 = Get Date/Time In Seconds() -> (seconds since 1Jan1904=w254:timestamp)
                  n140 = Wait (ms)(milliseconds to wait=u32 100) -> ()  [unwired: 1 out]
                  n141 = To Double Precision Float(number=w254) -> (double precision float=w267:dbl)
                  n142 = Subtract(x=w267, y=w262) -> (x-y=w252:dbl)
                  n143 = local read "abort"() -> (w260:bool)
                  n144 = Subtract(x=w261, y=w252) -> (x-y=w251:dbl)
                  n145 = Not(x=w260) -> (.not. x?=w266:bool)
                  n146 = Greater Than 0?(x=w251) -> (x > 0?=w253:bool)
                  n147 = Format Into String(format string="%d", w251) -> (resulting string=w265:string)  [unwired: 2 in, 1 out]
                  n148 = And(x=w253, y=w266) -> (x .and. y?=w263:bool)
                  n149 = Concatenate Strings(w255, "\r\n", "Timer status: ", w265) -> (w259:string)
                  n150 = local write "STATUS 1"(w259) -> ()
                }
              }
              frame #1 {
                n151 = local read "abort"() -> (w269:bool)
                n152 = case shown="False" w269 {
                  tunnel: [w280 w410] -> w270
                  tunnel: w271 -> [w279 _]
                  tunnel: w272 -> [w278 _]
                  tunnel: [w276 w410] -> w273
                  tunnel: w274 -> [w277 _]
                  tunnel: [w275 w410] -> w268
                  frame False {
                    n153 = stacked-sequence {
                      seq-local: [w281 _ _] -> [_ w321 _]
                      seq-local: [w291 _ _] -> [_ _ w379]
                      seq-local: [w290 _ _] -> [_ _ w380]
                      tunnel: w277 -> [_ _ w385]
                      tunnel: w278 -> [_ _ w376]
                      tunnel: [_ _ w383] -> w280
                      tunnel: [_ _ w382] -> w276
                      tunnel: w279 -> [_ _ _]
                      tunnel: [w298 _ _] -> w275
                      frame #0 {
                        w293 = T2."Write Element" ("Action")
                        # "SMU data"
                        n154 = Get Date/Time String(want seconds? (F)=TRUE) -> (time string=w295:string)  [unwired: 2 in, 1 out]
                        n155 = local write "Last reading at:"(w295) -> ()
                        n156 = local write "STATUS 1"("Reading current ..." ("status")) -> ()
                        n157 = global read "QC_MeasurementSetup.vi" "Ris Measurement Parameters"() -> (w289:T7)
                        n158 = Unbundle By Name(w289) -> ("Bias Supply"=w283:refnum<class "SupplyControl.lvclass">, "Set Current Limit?"=w288:bool, "Current Limit [µA]"=w285:dbl, "Temperature Readout"=w287:enum16{"Read Arduino", "Enter manually"}, "Arduino"=w282:refnum<class "ArduinoControl.lvclass">)
                        n159 = case shown="\"Read Arduino\"" w287 {
                          tunnel: [w308 w314] -> w296
                          tunnel: [w305 w313] -> w292
                          tunnel: w282 -> [_ w312]
                          frame "Enter manually", Default {
                            n160 = local read "Temp."() -> (w310:dbl[])
                            n161 = local read "RH"() -> (w306:dbl[])
                            n162 = Index Array(array=w310, index=0) -> (element=w308:dbl)
                            n163 = Index Array(array=w306, index=0) -> (element=w305:dbl)
                          }
                          frame "Read Arduino" {
                            n164 = call "ArduinoRead.vi"("Arduino function"=enum16{"T/RH", "Interlock", "Edgesense"}."T/RH", "ArduinoControl in"=w312) -> ("rel. Humidity [%]"=w313:dbl, "Temperature [°C]"=w314:dbl)  [unwired: 4 in, 4 out]
                          }
                        }
                        n165 = Multiply(x=w285, y=1000.0) -> (x*y=w284:dbl)
                        n166 = call-dynamic "Supply_ReadCurrent.vi"("SupplyControl in"=w283) -> ("error out"=w290:errorcluster, "Current in nA"=w299:dbl, "SupplyControl out"=w291:refnum<class "SupplyControl.lvclass">)  [unwired: 8 in]
                        n167 = case shown="True" w288 {
                          tunnel: w299 -> [_ w319]
                          tunnel: w284 -> [_ w317]
                          tunnel: [FALSE w316] -> w298
                          frame False {
                          }
                          frame True {
                            n168 = Absolute Value(x=w319) -> (abs(x)=w318:dbl)
                            n169 = Greater?(x=w318, y=w317) -> (0:w316:bool)
                          }
                        }
                        n170 = local read "Current reading No."() -> (w281:u32)
                        n171 = local read "Current Volts:"() -> (w300:dbl)
                        n172 = call "RisData.vi"("Action"=w293, "Array No."=u32 1, "Array Size / Index"=w281, "Data IN"=w299) -> ()  [unwired: 1 in, 2 out]
                        n173 = call "RisData.vi"("Action"=w293, "Array No."=u32 3, "Array Size / Index"=w281, "Data IN"=w296) -> ()  [unwired: 1 in, 2 out]
                        n174 = call "RisData.vi"("Action"=w293, "Array No."=u32 4, "Array Size / Index"=w281, "Data IN"=w292) -> ()  [unwired: 1 in, 2 out]
                        n175 = call "RisData.vi"("Action"=w293, "Array No."=0, "Array Size / Index"=w281, "Data IN"=w300) -> ()  [unwired: 1 in, 2 out]
                      }
                      frame #1 {
                        n176 = global read "QC_MeasurementSetup.vi" "Ris Measurement Parameters"() -> (w340:T7)
                        n177 = local read "Current Volts:"() -> (w343:dbl)
                        n178 = Unbundle By Name(w340) -> ("SMU"=w339:refnum<class "SupplyControl.lvclass">, "Multimeter"=w338:refnum<class "MultimeterControl.lvclass">)
                        n179 = call "RintSweep.vi"("Action"=enum16{"Reset", "Measure"}."Measure", "MasterVoltage Supply in"=w339, "VoltmeterControl in"=w338, "No. of readouts"="No. of readouts", "Bias [V]"=w343, "Simulated data?"=FALSE) -> ("Sweep"=w347:i32[], "Applied Current [nA]"=w327:dbl[][][], "Induced Voltage [V]"=w328:dbl[][][], "Voltages OUT"=w330:dbl[], "Compliance exceeded?"=w337:bool)  [unwired: 2 in, 3 out]
                        n180 = property on="Bias On/Off:" class="Bool (strict)"("Blinking"=w337) -> ()  [unwired: 2 in, 2 out]
                        n181 = local write "Ris SMU Current [nA]"(w327) -> ()
                        n182 = Array Size(array=w330) -> (size(s)=w345:i32)
                        n183 = Array Size(array=w347) -> (size(s)=w346:i32)
                        n184 = local write "Ris induced Voltage [V]"(w328) -> ()
                        n185 = for {
                          N: w345 -> [_]
                          tunnel: "No. of readouts" -> [w365]
                          tunnel: w346 -> [w364]
                          tunnel: w327 -> [w363] mode=indexing
                          tunnel: w328 -> [w362] mode=indexing
                          tunnel: w347 -> [w358]
                          tunnel: [w353] -> w336 mode=indexing
                          tunnel: [w352] -> w333 mode=indexing
                          tunnel: [w354] -> w326 mode=indexing
                          tunnel: [w354] -> w322
                          tunnel: [w349] -> w335 mode=indexing
                          tunnel: [w348] -> w332 mode=indexing
                          w361 = T9 0 items=["Least Square", "Least Absolute Residual", "Bisquare"] ("method")
                          w360 = T9 0 items=["Least Square", "Least Absolute Residual", "Bisquare"] ("method")
                          n186 = for {
                            N: w364 -> [_]
                            tunnel: w365 -> [_]
                            tunnel: w363 -> [w371] mode=indexing
                            tunnel: w362 -> [w370] mode=indexing
                            tunnel: [w369] -> w359 mode=indexing
                            tunnel: [w368] -> w357 mode=indexing
                            tunnel: [w367] -> w350 mode=indexing
                            tunnel: [w366] -> w351 mode=indexing
                            n187 = call <vilib>:"Std Deviation and Variance.vi"("X"=w371) -> ("mean"=w369:dbl, "standard deviation"=w367:dbl)  [unwired: 1 in, 1 out]
                            n188 = call <vilib>:"Std Deviation and Variance.vi"("X"=w370) -> ("mean"=w368:dbl, "standard deviation"=w366:dbl)  [unwired: 1 in, 1 out]
                          }
                          n189 = call <vilib>:"Linear Fit.vi"("Y"=w359, "X"=w358, "method"=w361) -> ("slope"=w355:dbl)  [unwired: 8 in, 4 out]
                          n190 = call <vilib>:"Linear Fit.vi"("Y"=w357, "X"=w358, "method"=w360) -> ("slope"=w356:dbl)  [unwired: 8 in, 4 out]
                          n191 = Bundle("Sweep"=w358, w359) -> (w353:cluster{"Sweep":i32[], dbl[]})  [unwired: 1 in]
                          n192 = Bundle("Sweep"=w358, w357) -> (w352:cluster{"Sweep":i32[], dbl[]})  [unwired: 1 in]
                          n193 = formula code="y=1e9/(x1*x2);"("x1"=w355, "x2"=w356) -> ("y"=w354:dbl)
                          n194 = call "XYerrorbars.vi"("XY plot"=w353, "Yerror"=w350) -> ("Y error bars"=w349:cluster{dbl[], dbl[]})  [unwired: 6 in, 2 out]
                          n195 = call "XYerrorbars.vi"("XY plot"=w352, "Yerror"=w351) -> ("Y error bars"=w348:cluster{dbl[], dbl[]})  [unwired: 6 in, 2 out]
                        }
                        n196 = Absolute Value(x=w330) -> (abs(x)=w329:dbl[])
                        n197 = Build Array (concatenate)(w336, w335) -> (w334:cluster{"Sweep":dbl[], dbl[]}[])
                        n198 = Build Array (concatenate)(w333, w332) -> (w331:cluster{"Sweep":dbl[], dbl[]}[])
                        n199 = Bundle(w329, w326) -> (w325:cluster{dbl[], dbl[]})  [unwired: 1 in]
                        n200 = Increment(x=w321) -> (x+1=w320:u32)
                        n201 = call "RisData.vi"("Action"=T2."Write Element", "Array No."=2, "Array Size / Index"=w321, "Data IN"=w322) -> ()  [unwired: 1 in, 2 out]
                        n202 = local write "Imgraph"(w334) -> ()
                        n203 = local write "Vigraph"(w331) -> ()
                        n204 = local write "Risgraph"(w325) -> ()
                        n205 = local write "Current reading No."(w320) -> ()
                      }
                      frame #2 {
                        # "Increment volts and check for end of loop"
                        n206 = local read "positive ramp?"() -> (w381:bool)
                        n207 = local read "Current Volts:"() -> (w377:dbl)
                        n208 = case shown="True" w381 {
                          tunnel: w376 -> [w388 w392]
                          tunnel: w385 -> [w389 w395]
                          tunnel: [w387 w394] -> w372
                          tunnel: [w386 w391] -> w384
                          tunnel: w377 -> [w390 w393]
                          frame False {
                            n209 = Subtract(x=w390, y=w389) -> (x-y=w386:dbl)
                            n210 = Greater Or Equal?(x=w386, y=w388) -> (x >= y?=w387:bool)
                          }
                          frame True {
                            n211 = Add(x=w393, y=w395) -> (x+y=w391:dbl)
                            n212 = Less Or Equal?(x=w391, y=w392) -> (x <= y?=w394:bool)
                          }
                        }
                        n213 = Quotient & Remainder(x=w377, y=w376) -> (x-y*floor(x/y)=w378:dbl, floor(x/y)=w375:dbl)
                        n214 = Not Equal To 0?(x=w378) -> (x != 0?=w373:bool)
                        n215 = Equal To 0?(x=w375) -> (x = 0?=w374:bool)
                        n216 = Or(x=w373, y=w374) -> ()  [unwired: 1 out]
                        n217 = case shown="True" w372 {
                          tunnel: w384 -> [_ w406]
                          tunnel: [TRUE FALSE] -> w383
                          tunnel: [FALSE w407] -> w382
                          tunnel: w377 -> [_ w404]
                          tunnel: w380 -> [_ w403]
                          tunnel: w379 -> [_ w402]
                          frame False {
                          }
                          frame True {
                            n218 = local read "step [V]"() -> (w400:dbl)
                            n219 = call "SupplyRamp.vi"("error in"=w403, "Requested Voltage"=w406, "Step Size"=w400, "Step Delay"=100, "Supply IN"=w402, "Starting Voltage"=w404) -> ("error out"=w398:errorcluster, "Compliance exceeded"=w407:bool, "Current Voltage"=w401:dbl)  [unwired: 2 in, 1 out]
                            n220 = case shown="No Error" w398 {
                              tunnel: w401 -> [w409 _]
                              frame No Error {
                                n221 = local write "Current Volts:"(w409) -> ()
                              }
                              frame Error {
                              }
                            }
                            n222 = property on="Bias On/Off:" class="Bool (strict)"("Blinking"=w407) -> ()  [unwired: 2 in, 2 out]
                            n223 = local write "STATUS 1"("Incrementing volts.") -> ()
                          }
                        }
                      }
                    }
                  }
                  frame True {
                    w410 = FALSE
                  }
                }
              }
            }
            n224 = case shown="True" w233 {
              frame False {
              }
              frame True {
                n225 = property on="Bias On/Off:" class="Bool (strict)"("Blinking"=TRUE) -> ()  [unwired: 2 in, 2 out]
              }
            }
            n226 = Build Array(w235, w233, "abort", w234) -> (w239:bool[])
            n227 = Or Array Elements(Boolean array=w239) -> (logical OR=w241:bool)
            n228 = Not(x=w241) -> (.not. x?=w240:bool)
          }
        }
        frame True {
          w412 = FALSE
          # "compliance was exceeded when first voltage applied."
          # "Flag compliance as reason for end of run"
          n229 = local write "STATUS 1"("Run aborted - compliance exceeded.") -> ()
          n230 = Build Array(w412, TRUE, w412, w412) -> (w413:bool[])
        }
      }
      n231 = Search 1D Array(1D array=w224, element=TRUE) -> (index of element=w222:i32)  [unwired: 1 in]
      n232 = Increment(x=w222) -> (x+1=w221:i32)
      n233 = case shown="2" w221 {
        tunnel: ["" "Run ended normally" "Compliance exceeded" "Run aborted - by user" "Run aborted - Ilimit exceeded"] -> w216
        frame ..0 {
        }
        frame 1 {
        }
        frame 2 {
          # "Determine reason for end of run."
        }
        frame 3 {
        }
        frame 4.. {
        }
      }
      n234 = global read "QC_RunInformation.vi" "Run info"() -> (w220:T5)
      n235 = Bundle By Name(cluster=w220, "End of Run comment:"=w216) -> (w215:T5)
      n236 = Concatenate Strings(w216, "\r\n", "RAMPING DOWN VOLTS") -> (w219:string)
      n237 = global write "QC_RunInformation.vi" "Run info"(w215) -> ()
      n238 = local write "STATUS 1"(w219) -> ()
    }
    frame #4 {
      n239 = stacked-sequence {
        frame #0 {
          # "Tie up loose ends. Set volts to zero and switch to standby"
          # "Ramp down volts now"
          n240 = global read "QC_MeasurementSetup.vi" "Ris Measurement Parameters"() -> (w421:T7)
          n241 = Unbundle By Name(w421) -> ("SMU"=w417:refnum<class "SupplyControl.lvclass">, "Bias Supply"=w418:refnum<class "SupplyControl.lvclass">, "Ramp down steps [V]"=w420:dbl, "Ramp down Interval [s]"=w419:i32, "Multimeter"=w431:refnum<class "MultimeterControl.lvclass">, "Switching"=w432:refnum<class "Switching.lvclass">, "Matrix used?"=w433:bool)
          n242 = Multiply(x=w419, y=1000) -> (x*y=w423:i32)
          n243 = local read "Current Volts:"() -> (w426:dbl)
          n244 = call-dynamic "Supply_Stby.vi"("SupplyControl in"=w417) -> ("error out"=w416:errorcluster)  [unwired: 9 in, 1 out]
          n245 = call "SupplyRamp.vi"("error in"=w416, "Requested Voltage"=0.0, "Step Size"=w420, "Step Delay"=w423, "Supply IN"=w418, "Starting Voltage"=w426) -> ("error out"=w428:errorcluster, "Supply OUT"=w427:refnum<class "SupplyControl.lvclass">, "Current Voltage"=w424:dbl)  [unwired: 2 in, 1 out]
          n246 = local write "Current Volts:"(w424) -> ()
          n247 = call-dynamic "Supply_Stby.vi"("error in (no error)"=w428, "SupplyControl in"=w427) -> ("error out"=w429:errorcluster)  [unwired: 8 in, 1 out]
          n248 = call-dynamic "Multimeter_Reset.vi"("error in (no error)"=w429, "MultimeterControl in"=w431) -> ("error out"=w430:errorcluster)  [unwired: 8 in, 1 out]
          n249 = case shown="True" w433 {
            tunnel: w432 -> [_ w436]
            tunnel: w430 -> [_ w435]
            frame False {
            }
            frame True {
              n250 = call-dynamic "MatrixSwitch.vi"("error in (no error)"=w435, "Action"=T3."Reset", "Switching in"=w436) -> ()  [unwired: 6 in, 3 out]
            }
          }
        }
        frame #1 {
          w441 = 0
          n251 = local write "Bias On/Off:"(FALSE ("Visible")) -> ()
          n252 = local write "Current Volts:"(0.0 ("Current Volts:")) -> ()
          n253 = property on="Quit & Save" class="Bool"("DisabledEnum"=w441) -> ()  [unwired: 2 in, 2 out]
          n254 = property on="quit (no save)" class="Bool"("DisabledEnum"=w441) -> ()  [unwired: 2 in, 2 out]
          n255 = property on="abort" class="Bool (strict)"("DisabledEnum"=2) -> ()  [unwired: 2 in, 2 out]
          n256 = local write "STATUS 1"("Run finished. \nSave data?" ("STATUS 1")) -> ()
        }
        frame #2 {
          n257 = Current VI's Path() -> (path=w443:path)
          n258 = call "SaveJPEG.vi"("Test"="Ris", "File Path Control"=w443) -> ()  [unwired: 1 in, 2 out]
        }
      }
    }
    frame #5 {
      # "Loop and await decision on whether to save or junk data"
      n259 = while {
        tunnel: ["Quit & Save"] -> w454
        tunnel: ["quit (no save)"] -> w453
        stop <- w494 continue-if-true
        n260 = Not Or(1:"quit (no save)", 2:"Quit & Save") -> (0:w494:bool)
      }
      n261 = global read "QC_MeasurementSetup.vi" "Ris Measurement Parameters"() -> (w452:T7)
      n262 = Unbundle By Name(w452) -> ("Temperature Readout"=w451:enum16{"Read Arduino", "Enter manually"}, "Arduino"=w445:refnum<class "ArduinoControl.lvclass">)
      n263 = case shown="\"Read Arduino\"" w451 {
        tunnel: w445 -> [_ w492]
        frame "Enter manually", Default {
        }
        frame "Read Arduino" {
          n264 = call "ArduinoClose.vi"("ArduinoControl in"=w492) -> ()  [unwired: 9 in, 2 out]
        }
      }
      n265 = case shown="True" w453 {
        tunnel: [FALSE w497] -> w455
        frame False {
        }
        frame True {
          n266 = Two Button Dialog(message="Are you sure you don't want to save the data?", 1:"Quit" ("F button name (\"Cancel\")"), 2:"Save data" ("T button name (\"OK\")")) -> (T button?=w497:bool)
        }
      }
      n267 = Or(x=w454, y=w455) -> (x .or. y?=w450:bool)
      n268 = flat-sequence {
        tunnel: w450 -> [w477]
        tunnel: [w477] -> w446
        tunnel: [TRUE] -> w444
        frame #0 {
          w464 = "%010.2f"
          w469 = T2."Read Array" ("Action")
          n269 = local write "STATUS 1"("Saving Data ...") -> ()
          n270 = global read "QC_MeasurementSetup.vi" "Ris Measurement Parameters"() -> (w488:T7)
          n271 = call "RisData.vi"("Action"=w469, "Array No."=u32 1 ("Action")) -> ("Array OUT"=w482:dbl[])  [unwired: 3 in, 1 out]
          n272 = call "RisData.vi"("Action"=w469, "Array No."=u32 2 ("Action")) -> ("Array OUT"=w467:dbl[])  [unwired: 3 in, 1 out]
          n273 = call "RisData.vi"("Action"=w469, "Array No."=u32 0 ("Action")) -> ("Array OUT"=w461:dbl[])  [unwired: 3 in, 1 out]
          n274 = Build Array(w461, w482, w467) -> (w481:dbl[][])
          n275 = call "RisData.vi"("Action"=w469, "Array No."=u32 4 ("Action")) -> ("Array OUT"=w487:dbl[])  [unwired: 3 in, 1 out]
          n276 = call "RisData.vi"("Action"=w469, "Array No."=u32 3 ("Action")) -> ("Array OUT"=w462:dbl[])  [unwired: 3 in, 1 out]
          n277 = Unbundle By Name(w488) -> ("R_is Limit [MOhm]"=w471:dbl, "Number Of Steps"=w458:u32)
          n278 = call <vilib>:"Std Deviation and Variance.vi"("X"=w487) -> ("mean"=w478:dbl)  [unwired: 1 in, 2 out]
          n279 = call <vilib>:"Std Deviation and Variance.vi"("X"=w462) -> ("mean"=w479:dbl)  [unwired: 1 in, 2 out]
          n280 = Transpose 2D Array(2D array=w481) -> (transposed array=w480:dbl[][])
          n281 = local read "Ris induced Voltage [V]"() -> (w465:dbl[][][])
          n282 = local read "Ris SMU Current [nA]"() -> (w466:dbl[][][])
          n283 = call "ScanFeedback.vi"("measurement type"=T4."Ris") -> ("V breakdown"=w473:dbl)  [unwired: 4 in, 4 out]
          n284 = call "SaveDataFile.vi"("Data Array"=w480, "Temperature"=w479, "Humidity"=w478, "no. of arrays"=2, "Actual array lengths"=w458, "Array Titles"="Voltage[V] Current[nA] R_is[MOhm]", "Strip Segment"="", "Arrays format"=w464) -> ("Path + Filename OUT"=w463:string, "Error Out"=w460:errorcluster)  [unwired: 4 in, 2 out]
          n285 = Absolute Value(x=w473) -> (abs(x)=w472:dbl)
          n286 = Absolute Value(x=w471) -> (abs(x)=w470:dbl)
          n287 = call "SaveRisRawData.vi"("Filename"=w463, "Induced Voltage [V]"=w465, "Volts"=w461, "error in (no error)"=w460, "SMU Current [nA]"=w466, "Data formats"=w464, "Number of data points"=w458) -> ("error out"=w459:errorcluster)  [unwired: 3 in]
          n288 = Greater Or Equal?(x=w472, y=w470) -> (x >= y?=w474:bool)
          n289 = call "WriteLogFile.vi"("Automatic warning"="", "Data File"=w463, "Error In"=w459, "DUT passed?"=w474, "Value TechSpec criteria"=w473, "Files saved?"=w477) -> ()  [unwired: 5 in, 1 out]
        }
      }
      n290 = Select(t="Run finished.\nData saved." ("STATUS 1"), s=w446, f="Run finished.\nData not saved." ("STATUS 1")) -> (s? t:f=w449:string)
      n291 = local write "STATUS 1"(w449) -> ()
      "Done!" <- w444
    }
  }
